vi "Send Abort.vi"(8 "error in (no error)":errorcluster, 11 "DataProcessor in":refnum<class "DataProcessor.lvclass">) -> (0 "error out":errorcluster, 3 "DataProcessor out":refnum<class "DataProcessor.lvclass">)   [LabVIEW 2020, in "VolatusData.lvlib" / "DataProcessor.lvclass"]
uses:
  DataProcessor.lvclass
  DataProcessor.lvclass/DataProcessor.ctl
  Volatus/AbortAPI/AbortAPI.lvclass
  DataHandlerTask/DataHandlerTask.lvclass
  Volatus/Task/Task.lvclass
  C:/dev/lv20CE/relink/lv-volatus/VolatusData/DataHandlerTask/DataHandlerTask.lvclass
  C:/dev/lv20CE/relink/lv-volatus/Volatus/Task/Task.lvclass
  C:/Program Files (x86)/National Instruments/LabVIEW 2020/vi.lib/ActorFramework/Actor/Actor.lvclass
  C:/dev/lv20CE/relink/lv-volatus/Volatus/TaskStateHandler/TaskStateHandler.lvclass
  C:/dev/lv20CE/relink/lv-volatus/Volatus/VectoMessageHandler/VectoMessageHandler.lvclass
  C:/dev/lv20CE/relink/lv-volatus/Volatus/API Provider/API Provider.lvclass
  C:/dev/lv20CE/relink/lv-volatus/VolatusData/DataHandler/DataHandler.lvclass
  C:/dev/lv20CE/relink/lv-volatus/VolatusData/DataProcessor/DataProcessor.lvclass
  C:/dev/lv20CE/relink/lv-volatus/Volatus/Abortable/Abortable.lvclass
  C:/dev/lv20CE/relink/lv-volatus/Volatus/Reconfigurable/Reconfigurable.lvclass
  Volatus/Event Level.ctl
  Volatus/Volatus.lvlib
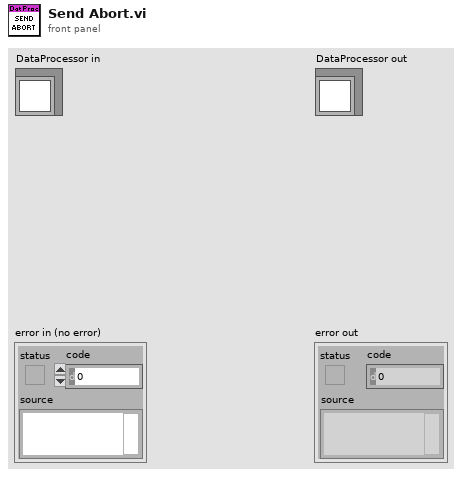
[diagram p1: front panel]
types:
  T1 = typedef "Volatus.lvlib/Event Level.ctl" = enum16{"Debug", "Info", "Warning", "Error"}
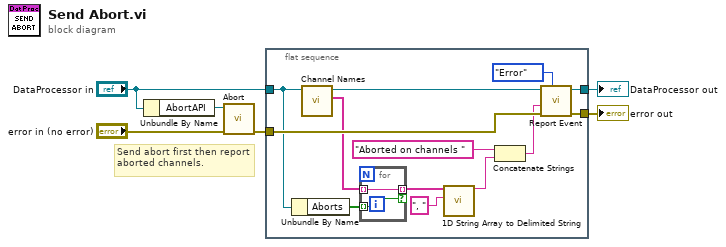
[diagram p0: block diagram]
diagram:
  # "Send abort first then report aborted channels."
  n1 = Unbundle By Name("DataProcessor in") -> ("AbortAPI"=w6:refnum<class "AbortAPI.lvclass">)
  n2 = call "Abort.vi"("error in (no error)"="error in (no error)", "AbortsAPI in"=w6) -> ("error out"=w5:errorcluster)  [unwired: 8 in, 1 out]
  n3 = flat-sequence {
    tunnel: w5 -> [w19]
    tunnel: "DataProcessor in" -> [w18]
    tunnel: [w11] -> w3
    tunnel: [w7] -> w1
    frame #0 {
      n4 = Unbundle By Name(w18) -> ("Aborts"=w17:bool[])
      n5 = call "Channel Names.vi"("DataHandlerTask in"=w18) -> ("Channel Names"=w16:string[], "DataHandlerTask out"=w13:refnum<class "DataProcessor.lvclass">)  [unwired: 8 in, 1 out]
      n6 = for {
        tunnel: w17 -> [w20] mode=indexing
        tunnel: w16 -> [w21] mode=indexing
        tunnel: [w21] -> w15 mode=indexing if=w20
      }
      n7 = call <vilib>:"1D String Array to Delimited String.vi"("delimiter"=", ", "string array"=w15) -> ("delimited string"=w9:string)  [unwired: 9 in]
      n8 = Concatenate Strings("Aborted on channels ", w9) -> (w8:string)
      n9 = call "Report Event.vi"("Level (Info)"=Event_Level."Error", "error in (no error)"=w19, "Message"=w8, "Task in"=w13) -> ("error out"=w7:errorcluster, "Task out"=w11:refnum<class "DataProcessor.lvclass">)  [unwired: 6 in]
    }
  }
  "error out" <- w1
  "DataProcessor out" <- w3
